vi "main drive.vi"(2 "error in (no error)":errorcluster, 3 "Stop? (Speeds = 0?)":bool, 4 "Array of Motor Speeds":dbl[](array[numeric]), 5 "VISA resource name":refnum<visa-resource-name>) -> (0 "error out":errorcluster, 1 "VISA resource name out":refnum<visa-resource-name>)   [LabVIEW 2018]
panel:
  # "This VI wraps the motor speeds, build msg and UART write VI's, and adds stop functionality\nby setting all of the speeds to zero when the Stop? button is triggered. Use this with the init\nmain VI."
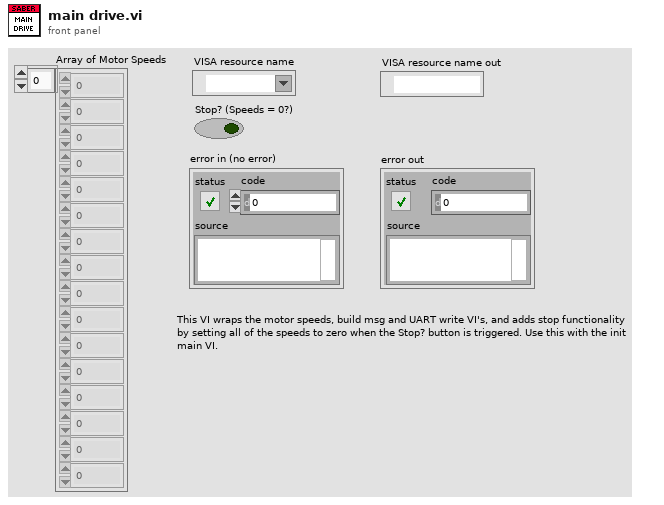
[diagram p1: front panel]
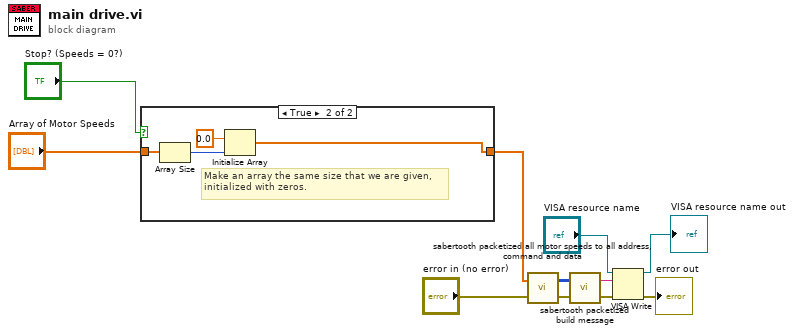
[diagram p0: block diagram]
diagram:
  n1 = case shown="True" "Stop? (Speeds = 0?)" {
    tunnel: "Array of Motor Speeds" -> [w12 w15]
    tunnel: [w12 w14] -> w1
    frame False {
    }
    frame True {
      # "Make an array the same size that we are given,\ninitialized with zeros."
      n2 = Array Size(array=w15) -> (size(s)=w13:i32)
      n3 = Initialize Array(0.0 ("element"), w13) -> (w14:dbl[])
    }
  }
  n4 = call "sabertooth packetized all motor speeds to all address, command and data.vi"("error in (no error)"="error in (no error)", "All Motor Speeds"=w1) -> ("error out"=w10:errorcluster, "Data to write"=w11:u8[][][])
  n5 = call "sabertooth packetized build message.vi"("error in (no error)"=w10, "Data to write"=w11) -> ("error out"=w9:errorcluster, "Uart Write Data"=w8:string)
  n6 = VISA Write(VISA resource name="VISA resource name", write buffer=w8, error in (no error)=w9) -> (VISA resource name out=→"VISA resource name out":refnum<visa-resource-name>, error out=→"error out":errorcluster)  [unwired: 1 out]
